vi "get status summary.vi"(1 "status code":u32 format="%x") -> (0 "flag names":string[](array[string]))   [LabVIEW 2024, in "atsj peakcan basic.lvlib"]
doc: "Converts a <b>status code</b> into individual <b>flag names</b>."
uses:
  atsj peakcan basic.lvlib
  status.ctl
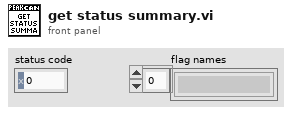
[diagram p1: front panel]
types:
  T1 = typedef "atsj peakcan basic.lvlib/status.ctl" = cluster{"xmtfull":bool, "overrun":bool, "buslight":bool, "busheavy":bool, "busoff":bool, "qrcvempty":bool, "qoverrun":bool, "qxmtfull":bool, "regtest":bool, "nodriver":bool, "hwinuse":bool, "netinuse":bool, "reserved1":bool, "resource":bool, "illparamtype":bool, "illparamval":bool, "unknown":bool, "illdata":bool, "buspassive":bool, "illmode":bool, "reserved2":bool, "reserved3":bool, "reserved4":bool, "reserved5":bool, "reserved6":bool, "caution":bool, "initialize":bool, "illoperation":bool, "reserved7":bool, "reserved8":bool, "reserved9":bool, "reserved10":bool}
  T2 = cluster{"Boolean array[0]":bool, "Boolean array[1]":bool, "Boolean array[2]":bool, "Boolean array[3]":bool, "Boolean array[4]":bool, "Boolean array[5]":bool, "Boolean array[6]":bool, "Boolean array[7]":bool, "Boolean array[8]":bool, "Boolean array[9]":bool, "Boolean array[10]":bool, "Boolean array[11]":bool, "Boolean array[12]":bool, "Boolean array[13]":bool, "Boolean array[14]":bool, "Boolean array[15]":bool, "Boolean array[16]":bool, "Boolean array[17]":bool, "Boolean array[18]":bool, "Boolean array[19]":bool, "Boolean array[20]":bool, "Boolean array[21]":bool, "Boolean array[22]":bool, "Boolean array[23]":bool, "Boolean array[24]":bool, "Boolean array[25]":bool, "Boolean array[26]":bool, "Boolean array[27]":bool, "Boolean array[28]":bool, "Boolean array[29]":bool, "Boolean array[30]":bool, "Boolean array[31]":bool}
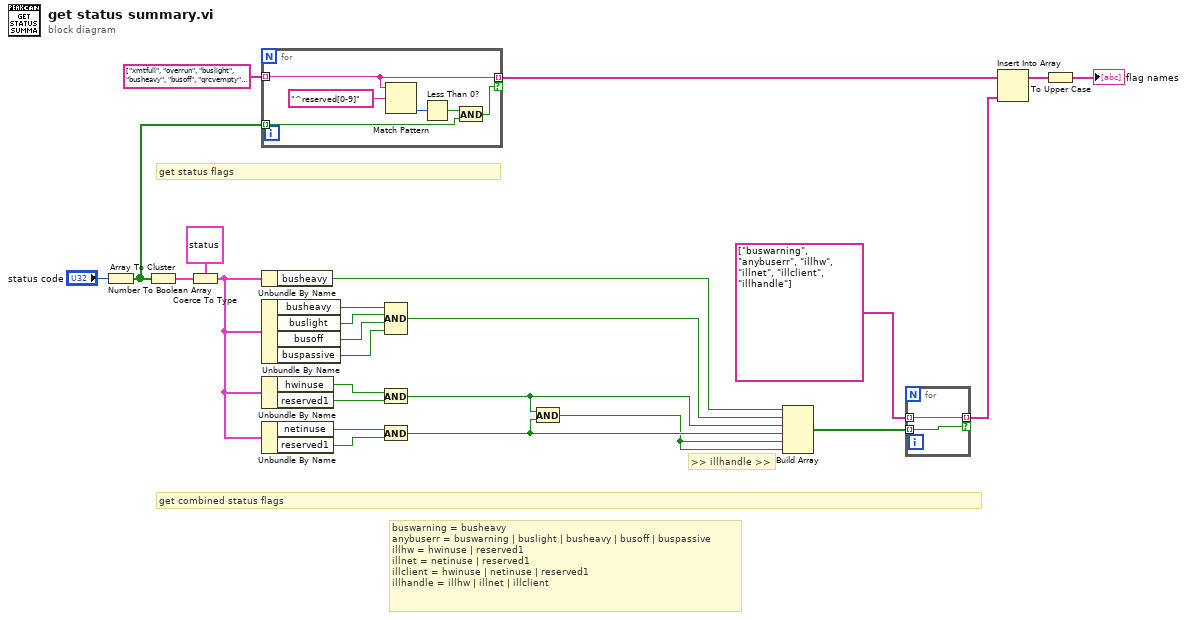
[diagram p0: block diagram]
diagram:
  # "get combined status flags"
  # "get status flags"
  # "buswarning = busheavy\nanybuserr = buswarning | buslight | busheavy | busoff | buspassive\nillhw = hwinuse | reserved1\nillnet = netinuse | reserved1\nillclient = hwinuse | netinuse | reserved1\nillhandle = illhw | illnet | illclient"
  # ">> illhandle >>"
  n1 = Number To Boolean Array(number="status code") -> (Boolean array=w7:bool[])
  n2 = Array To Cluster(array=w7) -> (cluster=w25:T2)
  n3 = Coerce To Type(0:w25, 1:T1 {"xmtfull"=FALSE, "overrun"=FALSE, "buslight"=FALSE, "busheavy"=FALSE, "busoff"=FALSE, "qrcvempty"=FALSE, "qoverrun"=FALSE, "qxmtfull"=FALSE, "regtest"=FALSE, "nodriver"=FALSE, "hwinuse"=FALSE, "netinuse"=FALSE, "reserved1"=FALSE, "resource"=FALSE, "illparamtype"=FALSE, "illparamval"=FALSE, "unknown"=FALSE, "illdata"=FALSE, "buspassive"=FALSE, "illmode"=FALSE, "reserved2"=FALSE, "reserved3"=FALSE, "reserved4"=FALSE, "reserved5"=FALSE, "reserved6"=FALSE, "caution"=FALSE, "initialize"=FALSE, "illoperation"=FALSE, "reserved7"=FALSE, "reserved8"=FALSE, "reserved9"=FALSE, "reserved10"=FALSE}) -> (2:w24:T1)
  n4 = for {
    tunnel: string[] ["xmtfull", "overrun", "buslight", "busheavy", "busoff", "qrcvempty", "qoverrun", "qxmtfull", "regtest", "nodriver", "hwinuse", "netinuse", "reserved1", "resource", "illparamtype", "illparamval", "unknown", "illdata", "buspassive", "illmode", "reserved2", "reserved3", "reserved4", "reserved5", "reserved6", "caution", "initialize", "illoperation", "reserved7", "reserved8", "reserved9", "reserved10"] -> [w31] mode=indexing
    tunnel: [w31] -> w6 mode=indexing if=w26
    tunnel: w7 -> [w27] mode=indexing
    n5 = Match Pattern(string=w31, regular expression="^reserved[0-9]") -> (offset past match=w29:i32)  [unwired: 1 in, 3 out]
    n6 = Less Than 0?(x=w29) -> (x < 0?=w28:bool)
    n7 = And(x=w28, y=w27) -> (x .and. y?=w26:bool)
  }
  n8 = Unbundle By Name(w24) -> ("busheavy"=w14:bool)
  n9 = Unbundle By Name(w24) -> ("busheavy"=w19:bool, "buslight"=w18:bool, "busoff"=w17:bool, "buspassive"=w16:bool)
  n10 = Unbundle By Name(w24) -> ("hwinuse"=w23:bool, "reserved1"=w22:bool)
  n11 = Unbundle By Name(w24) -> ("netinuse"=w21:bool, "reserved1"=w20:bool)
  n12 = And(x=w23, y=w22) -> (x .and. y?=w12:bool)
  n13 = And(x=w21, y=w20) -> (x .and. y?=w11:bool)
  n14 = Compound Arithmetic op=AND(w19, w18, w17, w16) -> (w13:bool)
  n15 = And(x=w12, y=w11) -> (x .and. y?=w10:bool)
  n16 = Build Array(w14, w13, w12, w11, w10, w10) -> (w9:bool[])
  n17 = for {
    tunnel: string[] ["buswarning", "anybuserr", "illhw", "illnet", "illclient", "illhandle"] -> [w33] mode=indexing
    tunnel: [w33] -> w5 mode=indexing if=w32
    tunnel: w9 -> [w32] mode=indexing
  }
  n18 = Insert Into Array(array=w6, new element=w5) -> (w4:string[])  [unwired: 1 in]
  n19 = To Upper Case(1:w4) -> (0:→"flag names":string[])
